vi "RootsPumpLCW_Status.vi"() -> (1 "n_ng":u8, 2 "values":T1)   [LabVIEW 2019]
uses:
  RootsPumpLCW_Global.vi
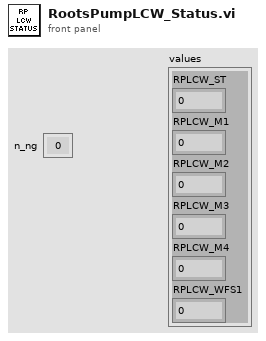
[diagram p1: front panel]
types:
  T1 = cluster{"RPLCW_ST":u32, "RPLCW_M1":dbl, "RPLCW_M2":dbl, "RPLCW_M3":dbl, "RPLCW_M4":dbl, "RPLCW_WFS1":dbl}
  T2 = enum32{"Bad", "Idle", "Run top level", "Running"}
  T3 = cluster{"MKS670_1000_ST":u32, "RPLCW_M1":dbl, "RPLCW_M2":dbl, "RPLCW_M3":dbl, "RPLCW_M4":dbl, "RPLCW_WFS1":dbl}
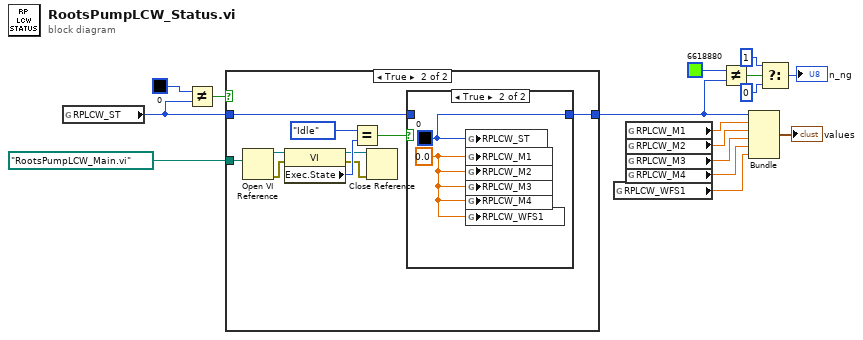
[diagram p0: block diagram]
diagram:
  n1 = global read "RootsPumpLCW_Global.vi" "RPLCW_ST"() -> (w7:u32)
  n2 = Not Equal?(x=u32 0 ("MKS670_1000_ST 2"), y=w7) -> (x != y?=w16:bool)
  n3 = case shown="True" w16 {
    tunnel: w7 -> [w17 w19]
    tunnel: [w17 w18] -> w13
    tunnel: path "RootsPumpLCW_Main.vi" ("vi path") -> [_ w20]
    frame False {
    }
    frame True {
      n4 = Open VI Reference(vi path=w20) -> (vi reference=w27:refnum<vi>, error out=w26:errorcluster)  [unwired: 5 in]
      n5 = property class="VI"(reference=w27, error in=w26) -> (reference out=w22:refnum<vi>, error out=w21:errorcluster, "Exec.State"=w24:T2)
      n6 = Equal?(x=T2."Idle" ("Execution:State"), y=w24) -> (x = y?=w25:bool)
      n7 = Close Reference(reference=w22, error in (no error)=w21) -> ()  [unwired: 1 out]
      n8 = case shown="True" w25 {
        tunnel: w19 -> [w28 _]
        tunnel: [w28 w30] -> w18
        frame False {
        }
        frame True {
          w29 = 0.0 ("MKS670_1000_P")
          w30 = u32 0 ("MKS670_1000_ST")
          n9 = global write "RootsPumpLCW_Global.vi" "RPLCW_ST"(w30) -> ()
          n10 = global write "RootsPumpLCW_Global.vi" "RPLCW_M1"(w29) -> ()
          n11 = global write "RootsPumpLCW_Global.vi" "RPLCW_M2"(w29) -> ()
          n12 = global write "RootsPumpLCW_Global.vi" "RPLCW_M3"(w29) -> ()
          n13 = global write "RootsPumpLCW_Global.vi" "RPLCW_M4"(w29) -> ()
          n14 = global write "RootsPumpLCW_Global.vi" "RPLCW_WFS1"(w29) -> ()
        }
      }
    }
  }
  n15 = global read "RootsPumpLCW_Global.vi" "RPLCW_WFS1"() -> (w3:dbl)
  n16 = global read "RootsPumpLCW_Global.vi" "RPLCW_M1"() -> (w6:dbl)
  n17 = global read "RootsPumpLCW_Global.vi" "RPLCW_M2"() -> (w5:dbl)
  n18 = global read "RootsPumpLCW_Global.vi" "RPLCW_M3"() -> (w4:dbl)
  n19 = global read "RootsPumpLCW_Global.vi" "RPLCW_M4"() -> (w2:dbl)
  n20 = Not Equal?(x=u32 6618880 ("MKS670_1000_ST 2"), y=w13) -> (x != y?=w11:bool)
  n21 = Bundle("MKS670_1000_ST"=w13, "RPLCW_M1"=w6, "RPLCW_M2"=w5, "RPLCW_M3"=w4, "RPLCW_M4"=w2, "RPLCW_WFS1"=w3) -> (→"values":T3)  [unwired: 1 in]
  n22 = Select(t=u8 1 ("n_ng"), s=w11, f=u8 0 ("n_ng")) -> (s? t:f=→"n_ng":u8)
